vi "GetFilePath.vi"(0 "path":path=path "C:/Data/Junk", 7 "file name":string="tst", 11 "frame number":u32) -> (4 "complete path":path=path "C:/Data/Junk", 8 "final path C":string, 15 "final path LV":string)   [LabVIEW 2016]
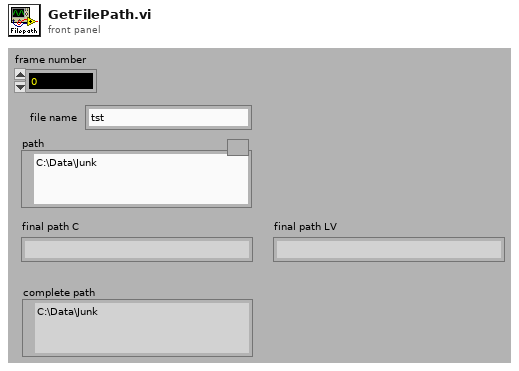
[diagram p1: front panel]
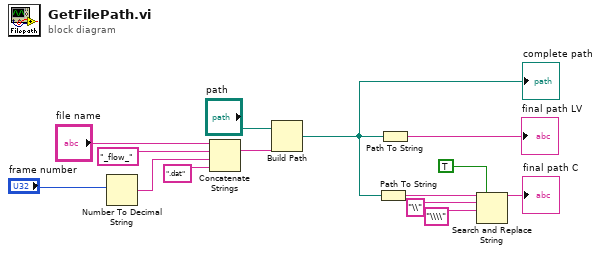
[diagram p0: block diagram]
diagram:
  n1 = Number To Decimal String(number="frame number") -> (decimal integer string=w10:string)  [unwired: 1 in]
  n2 = Concatenate Strings("file name", "_flow_", w10, ".dat") -> (w9:string)
  n3 = Build Path(base path="path", name or relative path=w9) -> (appended path=w1:path)
  "complete path" <- w1
  n4 = Path To String(path=w1) -> (string=w7:string)
  n5 = Path To String(path=w1) -> (string=→"final path LV":string)
  n6 = Search and Replace String(replace all?=TRUE, input string=w7, search string="\\", replace string="\\\\") -> (result string=→"final path C":string)  [unwired: 4 in, 3 out]
